vi "Global Variables v1.vi"() -> ()   [LabVIEW 2016]
panel:
  in  "go near RCM":bool
  in  "Irrigate?":bool
  in  "Start over tracking?":bool
  out "Last loop index":i32
  out "refractive index":dbl=1.35
  in  "joint limits":dbl[][](array[numeric])=[[-10.0, 35.0], [-35.0, 35.0], [0.1, 10.0], [-40.0, 40.0]]
  in  "assign pt out of bound":bool
  out "z monitor":dbl
  out "assign pt (x,y,z)":dbl[](array[numeric])
  in  "lock robot":bool
  out "OCT Z init Posit":dbl
  out "z rot axis":dbl
  out "z dist thld":dbl[](array[numeric])
  out "vac extremum":dbl[](array[numeric])
  in  "current run no.":u8
  out "assign point":dbl[](array[numeric])
  in  "assign pt reroute finished":bool
  in  "go to assign pt":bool
  in  "speed":u16(ring) items=["1x", "0.5x", "0.2x", "0.1x", "PAUSE"]
  in  "no. of runs":u8
  out "deform array":dbl[](array[numeric])
  in  "reset joystick":bool
  out "remote ctrl source":u16
  out "vacuum slide":i8
  out "max limit [mmHg]":dbl
  out "finished late counts":u16
  out "Accurus cluster":T1
  in  "L3 go home":bool
  out "OCT Z out Posit":dbl
  out "OCT Z cmd Posit":dbl
  out "Stage cmd Posit":dbl[](array[numeric])
  out "L1 to L4 cmd Posit":dbl[](array[numeric])
  out "L1 to L4 out Posit":dbl[](array[numeric])
  out "Stage out Posit":dbl[](array[numeric])
  in  "stop accurus":bool
  in  "state changing":bool
  out "state flag array":bool[](array[boolean])
  in  "program stop":bool
  # "homing finished"
  # "tracking initialization finished"
  # "trajecoty loading finished"
  # "tool engaged"
  # "tracking finshed"
  # "M/S initialization finished"
  # "button 1"
  # "button 2"
  # "button 3"
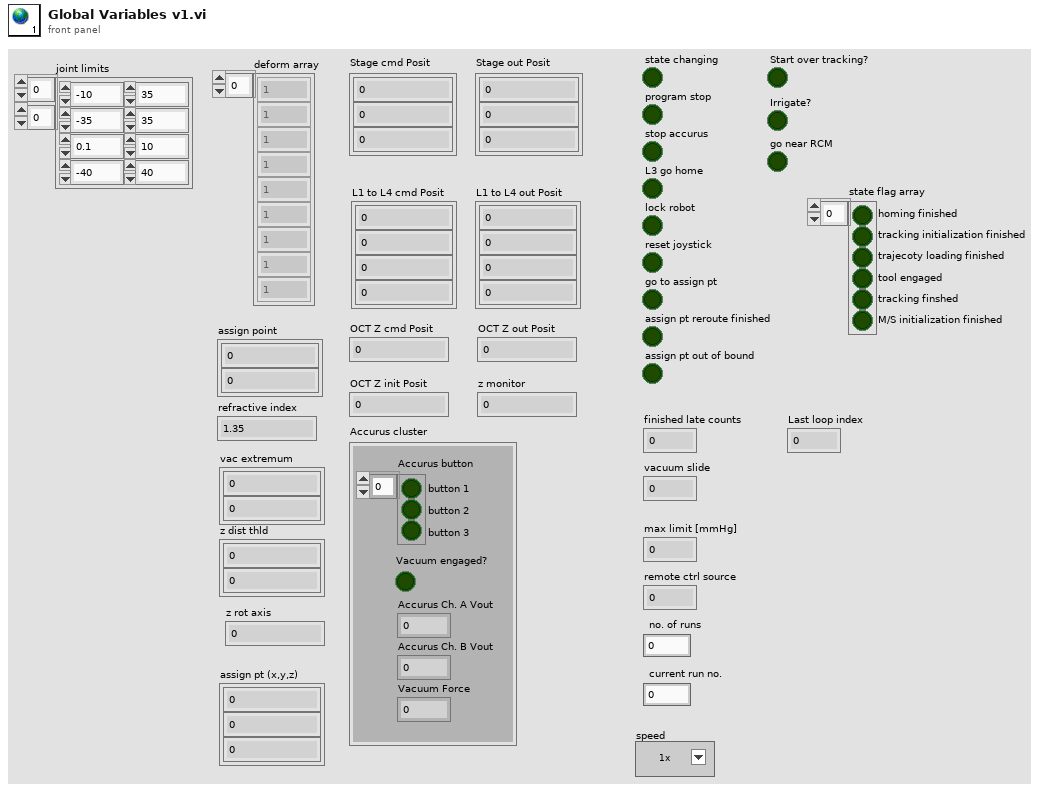
[diagram p1: front panel]
types:
  T1 = cluster{"Accurus button":bool[], "Vacuum engaged?":bool, "Vacuum Force":i32, "Accurus Ch. A Vout":dbl, "Accurus Ch. B Vout":dbl}
diagram:
